vi "4461 - Create Reference Waveforms.vi"(8 "error in (no error)":errorcluster, 9 "sampling info":cluster{"Fs":dbl, "#s":dbl}={"Fs"=1000.0, "#s"=1000.0} {"Fs" format="%.2p"}, 10 "reset signal":bool, 11 "Lockin":T1={"REF f (Hz)"=[13.0, 13.0, 13.0, 13.0, 13.0, 13.0, 13.0, 13.0], "REF phi (deg)"=[0.0, 0.0, 0.0, 0.0, 0.0, 0.0, 0.0, 0.0]} {"REF phi (deg)" format="%#_3g"}) -> (0 "error out":errorcluster, 1 "phase out":dbl[](array[numeric]), 2 "AO Array":waveform(dbl)[](array[waveform]), 3 "Lockin 2":T1={"REF f (Hz)"=[13.0, 13.0, 13.0, 13.0, 13.0, 13.0, 13.0, 13.0], "REF phi (deg)"=[0.0, 0.0, 0.0, 0.0, 0.0, 0.0, 0.0, 0.0]} {"REF phi (deg)" format="%#_3g"})   [LabVIEW 2013]
uses:
  <vilib>/Analysis/2dsp.llb/Decimate (single shot).vi
  <vilib>/Analysis/2dsp.llb/Decimate (single shot, DBL).vi
  <vilib>/Utility/error.llb/Error Cluster From Error Code.vi
  <vilib>/measure/NI_MABase.lvlib
panel:
  out "Waveform Graph 2":waveform(dbl)[](graph)=[{"t0"=timestamp(0 s since 1904-01-01), "dt"=4.8828125e-06, "Y"=array[20480 elements]}, {"t0"=timestamp(0 s since 1904-01-01), "dt"=4.8828125e-06, "Y"=array[20480 elements]}, {"t0"=timestamp(0 s since 1904-01-01), "dt"=4.8828125e-06, "Y"=array[20480 elements]}, {"t0"=timestamp(0 s since 1904-01-01), "dt"=4.8828125e-06, "Y"=array[20480 elements]}, {"t0"=timestamp(0 s since 1904-01-01), "dt"=4.8828125e-06, "Y"=array[20480 elements]}, {"t0"=timestamp(0 s since 1904-01-01), "dt"=4.8828125e-06, "Y"=array[20480 elements]}, {"t0"=timestamp(0 s since 1904-01-01), "dt"=4.8828125e-06, "Y"=array[20480 elements]}, {"t0"=timestamp(0 s since 1904-01-01), "dt"=4.8828125e-06, "Y"=array[20480 elements]}]
  out "Numeric":i32
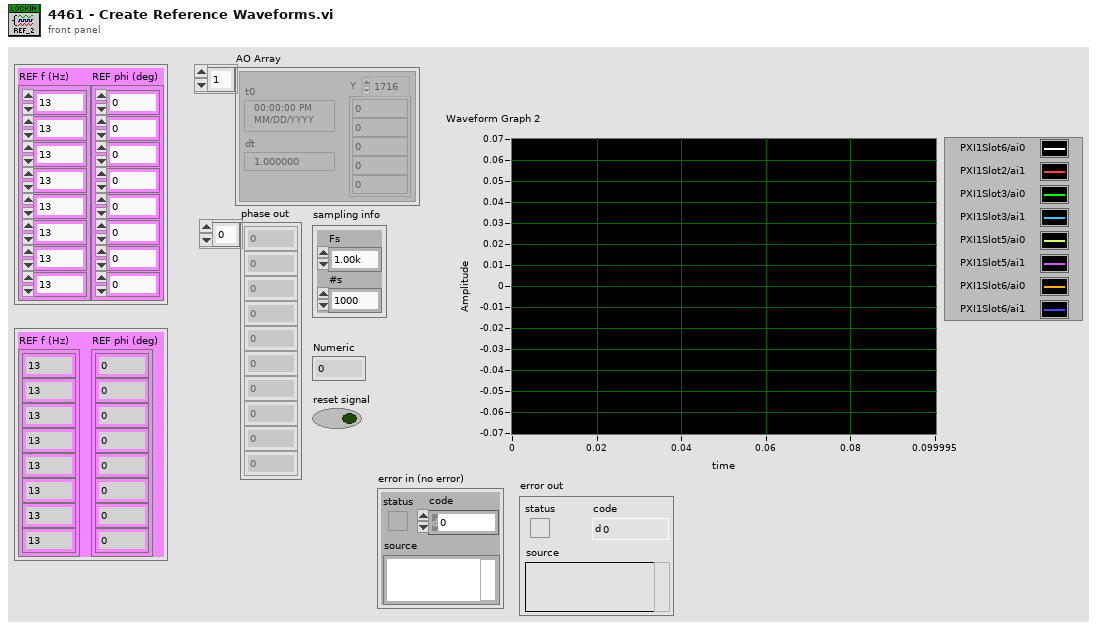
[diagram p1: front panel]
types:
  T1 = cluster{"REF f (Hz)":dbl[], "REF phi (deg)":dbl[]}
  T2 = enum16{"Sine Wave", "Triangle Wave", "Square Wave", "Sawtooth Wave"}
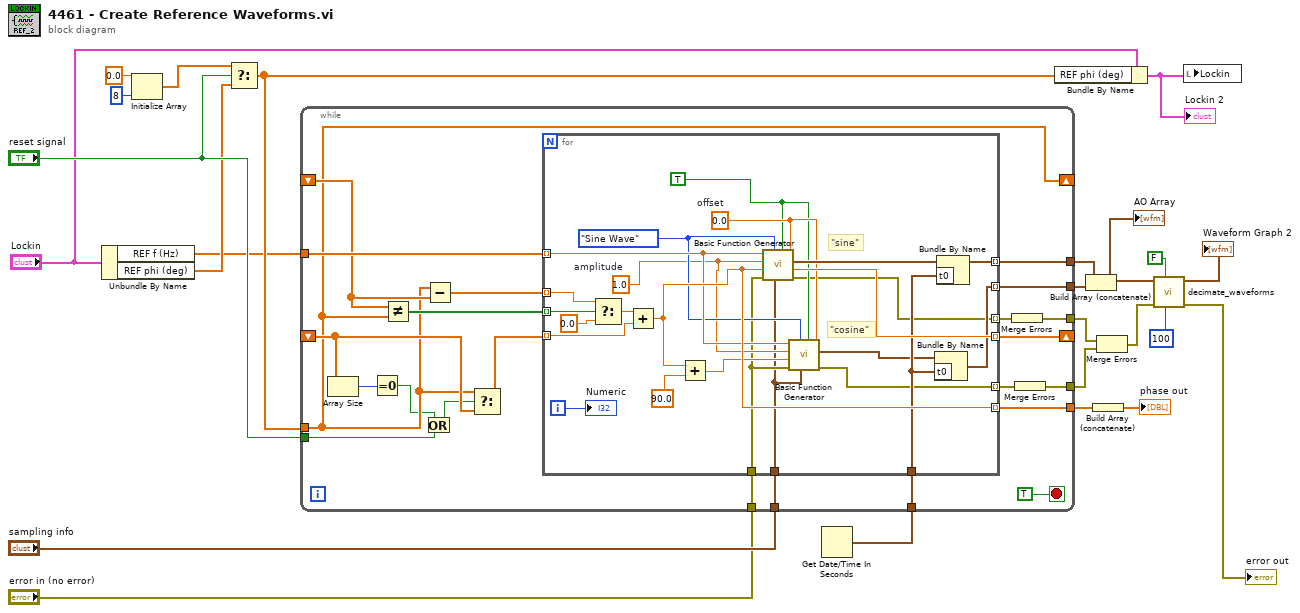
[diagram p0: block diagram]
diagram:
  n1 = Unbundle By Name("Lockin") -> ("REF f (Hz)"=w12:dbl[], "REF phi (deg)"=w13:dbl[])
  n2 = Initialize Array(0.0 ("element"), 8 ("dimension size")) -> (w20:dbl[])
  n3 = Select(t=w20, s="reset signal", f=w13) -> (s? t:f=w19:dbl[])
  n4 = Get Date/Time In Seconds() -> (seconds since 1Jan1904=w21:timestamp)
  n5 = while {
    tunnel: "sampling info" -> [w47]
    tunnel: [w46] -> w14
    tunnel: w19 -> [w35]
    tunnel: w12 -> [w45]
    shift-right: [w35] -> _
    shift-left: _ -> [w42]
    shift-right: [w40] -> _
    shift-left: _ -> [w37]
    tunnel: w21 -> [w38]
    tunnel: "reset signal" -> [w32]
    tunnel: [w31] -> w17
    tunnel: [w30] -> w15
    tunnel: "error in (no error)" -> [w29]
    tunnel: [w27] -> w3
    tunnel: [w25] -> w4
    stop <- TRUE stop-if-true
    n6 = Array Size(array=w37) -> (size(s)=w36:i32)
    n7 = Equal To 0?(x=w36) -> (x = 0?=w33:bool)
    n8 = Not Equal?(x=w42, y=w35) -> (x != y?=w43:bool[])
    n9 = Or(x=w33, y=w32) -> (x .or. y?=w34:bool)
    n10 = Subtract(x=w35, y=w42) -> (x-y=w41:dbl[])
    n11 = Select(t=w35, s=w34, f=w37) -> (s? t:f=w39:dbl[])
    n12 = for {
      tunnel: w45 -> [w59] mode=indexing
      tunnel: [w70] -> w46 mode=indexing
      tunnel: w47 -> [w50]
      tunnel: w43 -> [w64] mode=indexing
      tunnel: w41 -> [w66] mode=indexing
      tunnel: [w62] -> w40 mode=indexing
      tunnel: w39 -> [w67] mode=indexing
      tunnel: w38 -> [w58]
      tunnel: [w61] -> w31 mode=indexing
      tunnel: [w56] -> w30 mode=indexing
      tunnel: w29 -> [w51]
      tunnel: [w49] -> w28 mode=indexing
      tunnel: [w48] -> w26 mode=indexing
      i -> [w63]
      w52 = TRUE ("reset signal")
      w54 = 0.0  # offset
      w55 = T2."Sine Wave" ("signal type")
      w53 = 1.0  # amplitude
      # "\"cosine\""
      # "\"sine\""
      n13 = Select(t=w66, s=w64, f=0.0) -> (s? t:f=w68:dbl)
      n14 = Add(x=w68, y=w67) -> (x+y=w61:dbl)
      n15 = Add(x=w61, y=90.0) -> (x+y=w60:dbl)
      n16 = call <vilib>:"Basic Function Generator.vi"("offset"=w54, "reset signal"=w52, "sampling info"=w50, "signal type"=w55, "error in (no error)"=w51, "phase"=w61, "amplitude"=w53, "frequency"=w59) -> ("error out"=w49:errorcluster, "phase out"=w62:dbl, "signal out"=w71:waveform(dbl))  [unwired: 1 in]
      n17 = call <vilib>:"Basic Function Generator.vi"("offset"=w54, "reset signal"=w52, "sampling info"=w50, "signal type"=w55, "error in (no error)"=w51, "phase"=w60, "amplitude"=w53, "frequency"=w59) -> ("error out"=w48:errorcluster, "signal out"=w57:waveform(dbl))  [unwired: 1 in, 1 out]
      n18 = Bundle By Name(cluster=w57, "t0"=w58) -> (w56:waveform(dbl))
      n19 = Bundle By Name(cluster=w71, "t0"=w58) -> (w70:waveform(dbl))
      "Numeric" <- w63
    }
    n20 = Merge Errors(w28) -> (w27:errorcluster)
    n21 = Merge Errors(w26) -> (w25:errorcluster)
  }
  n22 = Bundle By Name(cluster="Lockin", "REF phi (deg)"=w19) -> (w10:T1)
  "Lockin 2" <- w10
  n23 = Build Array (concatenate)(w14, w15) -> (w8:waveform(dbl)[])
  "AO Array" <- w8
  n24 = Build Array (concatenate)(w17) -> (→"phase out":dbl[])
  n25 = Merge Errors(w3, w4) -> (w2:errorcluster)
  n26 = call "decimate_waveforms.vi"("decimating factor"=100, "averaging"=FALSE, "error in (no error)"=w2, "Input Signal"=w8) -> ("error out"=→"error out":errorcluster, "Decimated Waveforms"=→"Waveform Graph 2":waveform(dbl)[])  [unwired: 6 in]
  n27 = local write "Lockin"(w10) -> ()
